vi "1.vi"() -> ()   [LabVIEW 2017]
panel:
  out "时间":string
  in  "停止":bool
  in  "启动":bool
  out "?":bool
  in  "时间选择":enum16{"6s", "10s", "20s"}(ring)
  # "倒计时器"
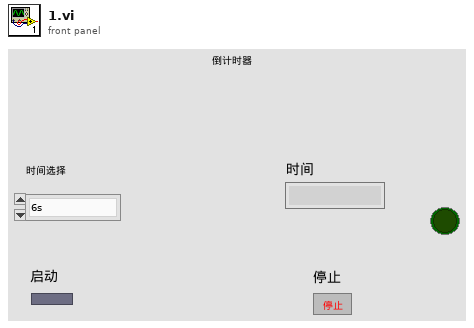
[diagram p1: front panel]
types:
  T1 = enum8{"Enabled", "Disabled", "Disabled and Grayed Out"}
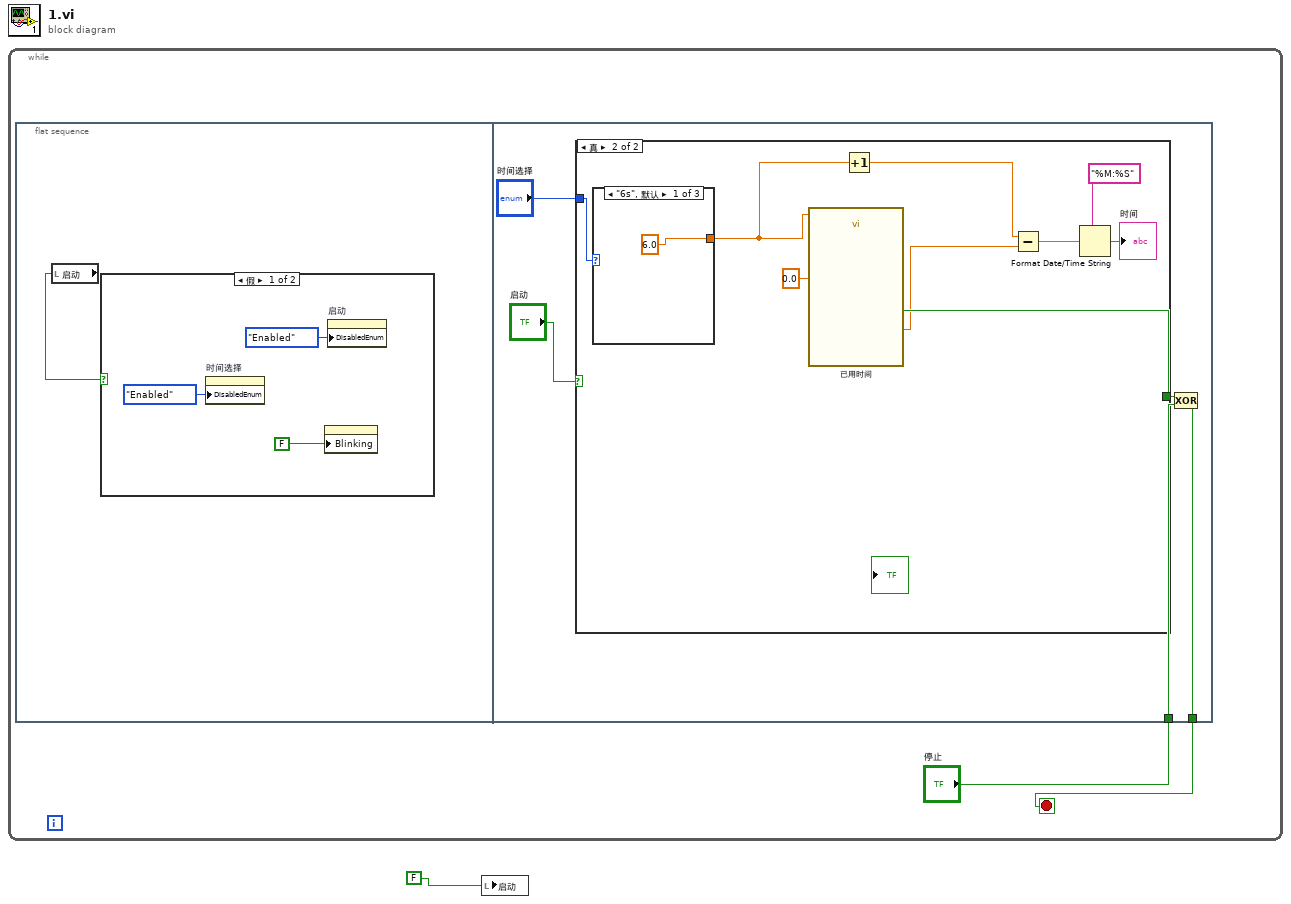
[diagram p0: block diagram]
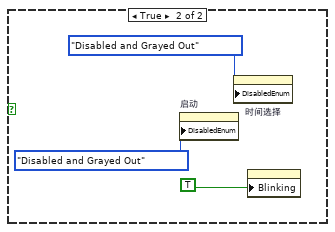
[diagram p2: hidden frame]
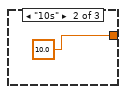
[diagram p4: hidden frame]
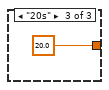
[diagram p5: hidden frame]
diagram:
  n1 = while {
    stop <- w2 stop-if-true
    n2 = flat-sequence {
      tunnel: "停止" -> [w13]
      tunnel: [w12] -> w2
      frame #0 {
        n3 = local read "启动"() -> (w4:bool)
        n4 = case shown="假" w4 {
          frame False {
            n5 = property on="时间选择" class="Enum (严格)"("DisabledEnum"=T1."Enabled" ("禁用")) -> ()  [unwired: 2 in, 2 out]
            n6 = property class="Bool (严格)"("Blinking"=FALSE) -> ()  [unwired: 2 in, 2 out]
            n7 = property on="启动" class="Bool (严格)"("DisabledEnum"=T1."Enabled" ("禁用")) -> ()  [unwired: 2 in, 2 out]
          }
          frame True {
            n8 = property on="启动" class="Bool (严格)"("DisabledEnum"=T1."Disabled and Grayed Out" ("禁用")) -> ()  [unwired: 2 in, 2 out]
            n9 = property on="时间选择" class="Enum (严格)"("DisabledEnum"=T1."Disabled and Grayed Out" ("禁用")) -> ()  [unwired: 2 in, 2 out]
            n10 = property class="Bool (严格)"("Blinking"=TRUE) -> ()  [unwired: 2 in, 2 out]
          }
        }
      }
      frame #1 {
        n11 = case shown="真" "启动" {
          tunnel: "时间选择" -> [_ w24]
          tunnel: [_ w23] -> w14
          frame False {
          }
          frame True {
            n12 = case shown="\"6s\", 默认" w24 {
              tunnel: [6.0 10.0 20.0] -> w19
              frame "6s", Default {
              }
              frame "10s" {
              }
              frame "20s" {
              }
            }
            n13 = call "已用时间"("Time Target (s)"=w19, "Set Start Time (s)"=0.0) -> ("Elapsed Time (s)"=w17:dbl, "Time has Elapsed"=w23:bool)  [unwired: 10 in, 6 out]
            n14 = Increment(x=w19) -> (x+1=w18:dbl)
            n15 = Subtract(x=w18, y=w17) -> (x-y=w16:dbl)
            n16 = Format Date/Time String(time format string (%c)="%M:%S" ("时间格式字符串(%c)"), seconds (now)=w16) -> (date/time string=→"时间":string)  [unwired: 1 in]
          }
        }
        n17 = Compound Arithmetic op=XOR(w14, w13) -> (w12:bool)
      }
    }
  }
  n18 = local write "启动"(FALSE) -> ()
